vi "_Save RT Table.vi"(4 "error in (no error)":errorcluster, 5 "Simulation":bool, 6 "Table":dbl[][](array[numeric]), 7 "key":string) -> (0 "error out":errorcluster)   [LabVIEW 2015]
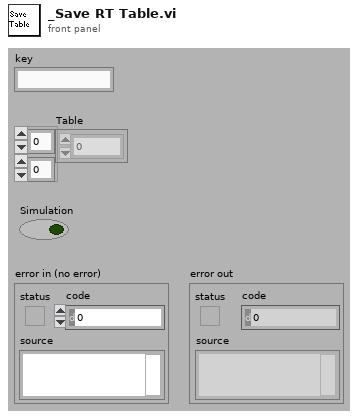
[diagram p1: front panel]
types:
  T1 = enum16{"open", "replace", "create", "open or create", "replace or create", "replace or create with confirmation"}
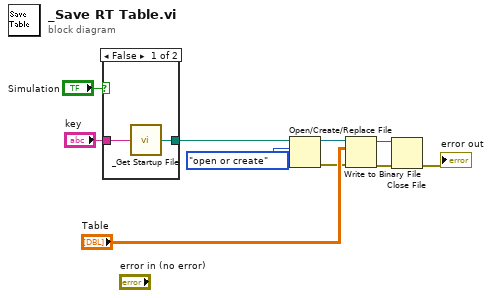
[diagram p0: block diagram]
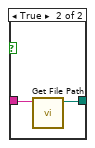
[diagram p2: hidden frame]
diagram:
  n1 = case shown="False" "Simulation" {
    tunnel: [w12 w13] -> w3
    tunnel: "key" -> [w11 w14]
    frame False {
      n2 = call "_Get Startup File.vi"("FileName"=w11) -> ("FilePath"=w12:path)
    }
    frame True {
      n3 = call "Get File Path.vi"("FileName"=w14) -> ("FilePath"=w13:path)  [unwired: 10 in]
    }
  }
  n4 = Open/Create/Replace File(file path (use dialog)=w3, operation (0:open)=T1."open or create") -> (refnum out=w2:refnum<file>, error out=w1:errorcluster)  [unwired: 4 in, 1 out]
  n5 = Write to Binary File(file (use dialog)=w2, data="Table", error in=w1) -> (refnum out=w9:refnum<file>, error out=w10:errorcluster)  [unwired: 4 out]
  n6 = Close File(refnum=w9, error in=w10) -> (error out=→"error out":errorcluster)  [unwired: 1 out]
